vi "AIN_CFG.vi"(0 "P-Channel":i8=1, 1 "VISA resource name":refnum<visa-resource-name>, 2 "N-Channel":i8, 3 "Gain":i8=1, 5 "nsamples":i8=1) -> (6 "VISA resource Salida":refnum<visa-resource-name>, 7 "AIN_data":u32, 8 "error out":errorcluster)   [LabVIEW 2011]
panel:
  out "unsigned byte array":u8[](array[numeric])
  out "Sent":u32
  out "Received":u32
  out "subarray":u8[](array[numeric])
  out "Read AIN command":u8[](array[numeric])
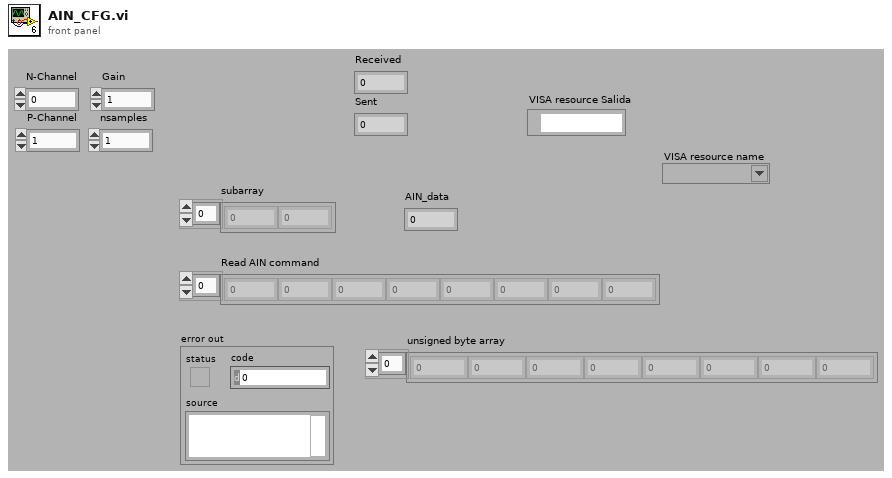
[diagram p1: front panel]
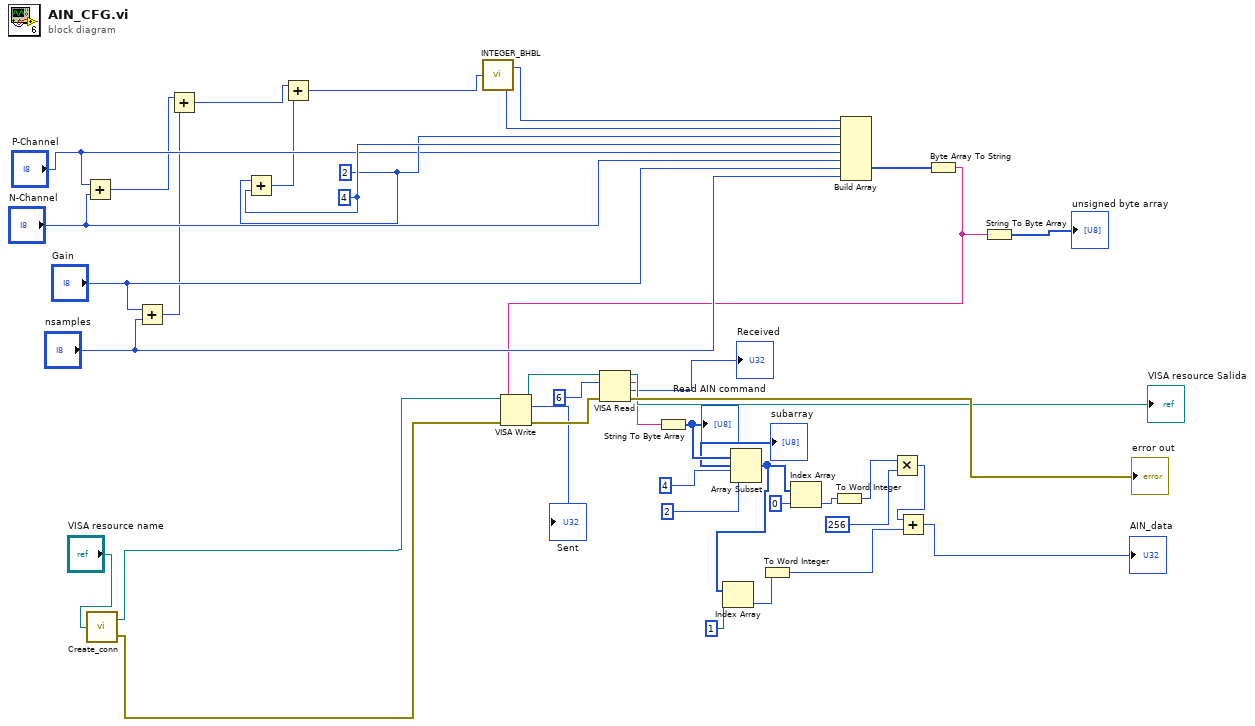
[diagram p0: block diagram]
diagram:
  w16 = i8 2 ("element")
  w17 = i8 4 ("element")
  n1 = Add(x="P-Channel", y="N-Channel") -> (x+y=w11:i8)
  n2 = call "Create_conn.vi"("VISA resourceINPUT"="VISA resource name") -> ("error out"=w2:errorcluster, "VISA resource name out"=w3:refnum<visa-resource-name>)
  n3 = Add(x="Gain", y="nsamples") -> (x+y=w10:i8)
  n4 = Add(x=w11, y=w10) -> (x+y=w9:i8)
  n5 = Add(x=w16, y=w17) -> (x+y=w8:i8)
  n6 = Add(x=w9, y=w8) -> (x+y=w7:i8)
  n7 = call "INTEGER_BHBL.vi"("int16"=w7) -> ("Lvalue"=w18:u8, "HValue"=w19:u8)
  n8 = Build Array(w19, w18, w16, w17, "P-Channel", "N-Channel", "Gain", "nsamples") -> (w22:u8[])
  n9 = Byte Array To String(unsigned byte array=w22) -> (string=w6:string)
  n10 = VISA Write(VISA resource name=w3, write buffer=w6, error in (no error)=w2) -> (VISA resource name out=w37:refnum<visa-resource-name>, return count=→"Sent":u32, error out=w40:errorcluster)
  n11 = VISA Read(VISA resource name=w37, byte count=u32 6, error in (no error)=w40) -> (VISA resource name out=→"VISA resource Salida":refnum<visa-resource-name>, read buffer=w36:string, return count=→"Received":u32, error out=→"error out":errorcluster)
  n12 = String To Byte Array(string=w36) -> (unsigned byte array=w34:u8[])
  "Read AIN command" <- w34
  n13 = Array Subset(array=w34, index=4, length=2) -> (w1:u8[])
  "subarray" <- w1
  n14 = Index Array(array=w1, index=1) -> (element=w27:u8)
  n15 = To Word Integer(number=w27) -> (16bit integer=w26:i16)
  n16 = Index Array(array=w1, index=0) -> (element=w28:u8)
  n17 = To Word Integer(number=w28) -> (16bit integer=w29:i16)
  n18 = Multiply(x=w29, y=i16 256) -> (x*y=w23:i16)
  n19 = Add(x=w23, y=w26) -> (x+y=→"AIN_data":i16)
  n20 = String To Byte Array(string=w6) -> (unsigned byte array=→"unsigned byte array":u8[])
